vi "Archive Config.vi"(8 "error in":errorcluster, 11 "Config Manager in":refnum<class "Config Manager Class.lvclass">) -> (0 "error out":errorcluster, 3 "Config Manager out":refnum<class "Config Manager Class.lvclass">)   [LabVIEW 2011, in "Config Manager Class.lvclass"]
uses:
  Config Manager Class.lvclass
  Config Manager Class.lvclass/Config Manager Class.ctl
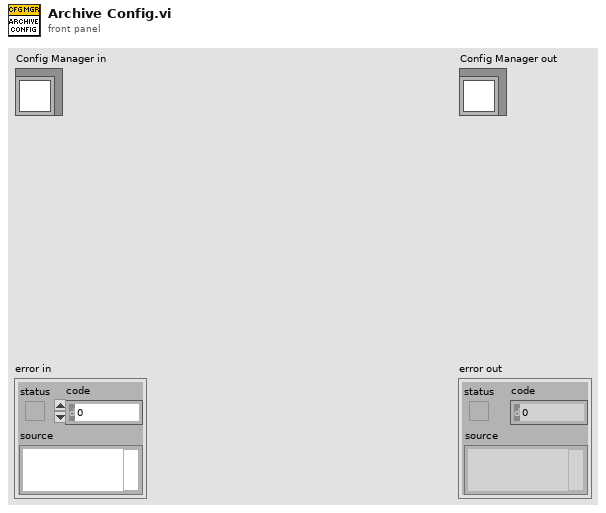
[diagram p1: front panel]
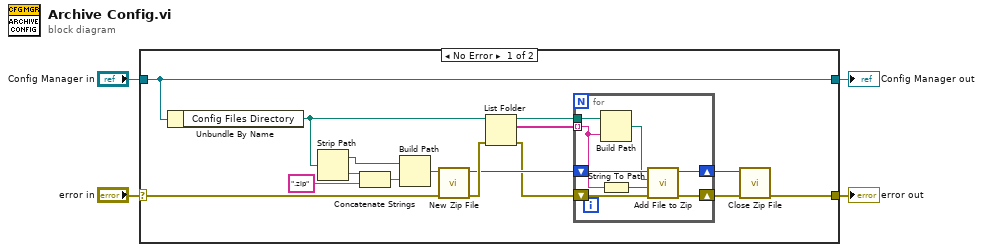
[diagram p0: block diagram]
diagram:
  n1 = case shown="No Error" "error in" {
    selector: "error in" -> [w14 w30]
    tunnel: [w5 w30] -> w3
    tunnel: [w20 w29] -> w1
    tunnel: "Config Manager in" -> [w20 w29]
    frame No Error {
      n2 = Unbundle By Name(w20) -> ("Config Files Directory"=w13:path)
      n3 = Strip Path(path=w13) -> (stripped path=w17:path, name=w19:string)
      n4 = Concatenate Strings(w19, ".zip" ("string")) -> (w16:string)
      n5 = Build Path(base path=w17, name or relative path=w16) -> (appended path=w15:path)
      n6 = call <vilib>:"New Zip File.vi"("error in (no error)"=w14, "target"=w15) -> ("error out"=w10:errorcluster, "zip file out"=w9:i64)  [unwired: 3 in, 1 out]
      n7 = List Folder(path=w13, error in=w10) -> (path out=w12:path, filenames=w11:string[], error out=w8:errorcluster)  [unwired: 2 in, 1 out]
      n8 = for {
        tunnel: w12 -> [w28]
        tunnel: w11 -> [w26] mode=indexing
        shift-right: [w22] -> w6
        shift-left: w8 -> [w23]
        shift-right: [w21] -> w7
        shift-left: w9 -> [w27]
        n9 = Build Path(base path=w28, name or relative path=w26) -> (appended path=w24:path)
        n10 = String To Path(string=w26) -> (path=w25:path)
        n11 = call <vilib>:"Add File to Zip.vi"("error in (no error)"=w23, "destination path in zip"=w25, "source file path"=w24, "zip file in"=w27) -> ("error out"=w22:errorcluster, "zip file out"=w21:i64)  [unwired: 6 in]
      }
      n12 = call <vilib>:"Close Zip File.vi"("error in (no error)"=w6, "zip file in"=w7) -> ("error out"=w5:errorcluster)  [unwired: 5 in]
    }
    frame Error {
    }
  }
  "error out" <- w3
  "Config Manager out" <- w1
